vi "IsStopped.vi"(8 "Error In":errorcluster, 11 "VISA resource name":refnum<visa-resource-name>) -> (0 "Error Out":errorcluster, 2 "IsStopped":bool, 3 "VISA resource name out":refnum<visa-resource-name>)   [LabVIEW 2019, in "Mark 10 TSTM-DC.lvlib"]
uses:
  Mark 10 TSTM-DC.lvlib
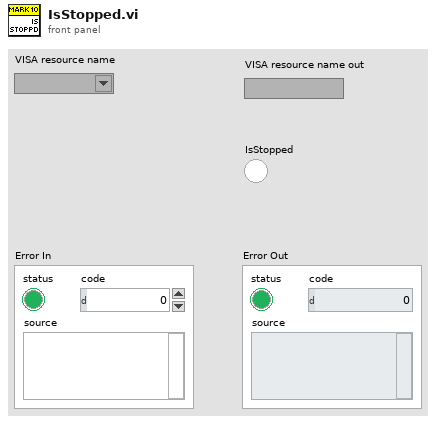
[diagram p1: front panel]
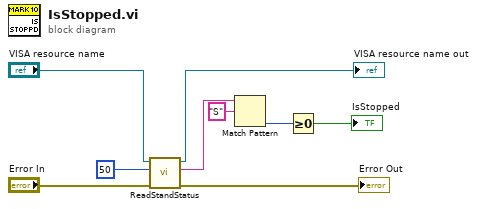
[diagram p0: block diagram]
diagram:
  n1 = call "ReadStandStatus.vi"("error in"="Error In", "milliseconds to wait"=u32 50, "VISA resource name"="VISA resource name") -> ("error out"=→"Error Out":errorcluster, "Status"=w4:string, "VISA resource name out"=→"VISA resource name out":refnum<visa-resource-name>)  [unwired: 6 in]
  n2 = Match Pattern(string=w4, regular expression="S") -> (offset past match=w2:i32)  [unwired: 1 in, 3 out]
  n3 = Greater Or Equal To 0?(x=w2) -> (x >= 0?=→"IsStopped":bool)
